vi "New Report Schema and Output Table Create.vi"() -> (0 "error out":errorcluster)   [LabVIEW 2023, in "HardwareAbstractionLayer_LVOOP.lvlib" / "Report.lvclass"]
uses:
  Report.lvclass
  Database/SQL Public VI/Control/DB Options.ctl
  <vilib>/Utility/error.llb/Trim Whitespace One-Sided.vi
  <userlib>/_OpenG.lib/array/array.llb/Filter 1D Array (String)__ogtk.vi
  Database/Database.lvclass
  Control/Action FGV.ctl
  Control/Result FGV Data.ctl
  <userlib>/_OpenG.lib/array/array.llb/openg_array.lvlib
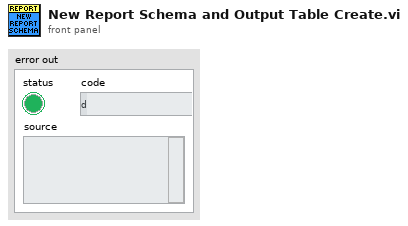
[diagram p1: front panel]
types:
  T1 = typedef "HardwareAbstractionLayer_LVOOP.lvlib/Database.lvclass/DB Options.ctl" = enum16{"Init", "Select Data", "Insert Data", "Update Data", "Delete Data", "Execute Query", "Create Schema", "Create Table", "List Tables", "List Columns", "Close"}
  T2 = typedef "HardwareAbstractionLayer_LVOOP.lvlib/Report.lvclass/Result FGV Data.ctl" = cluster{"Project Name":string, "Product Name":string, "Product Varient":string, "Test Name":string, "Test Phase":string, "Test Description":string, "Temp Chamber Name":string, "Schema":string, "Total No of Cycles":u32, "Current Cycle Number":u32, "Cycle Duration":u32, "Current Test Mode":string}
  T3 = typedef "HardwareAbstractionLayer_LVOOP.lvlib/Report.lvclass/Action FGV.ctl" = enum16{"Init", "Set Project Name", "Set Product Name", "Set Product Varient", "Set Test Name", "Set Test Phase", "Set Test Description", "Set Temp Chamber Name", "Set Cycle Duration", "Set Current Cycle Number", "Set Schema", "Set Total No Of Cycle", "Set Current Test Mode", "Set All Data", "Get All Data"}
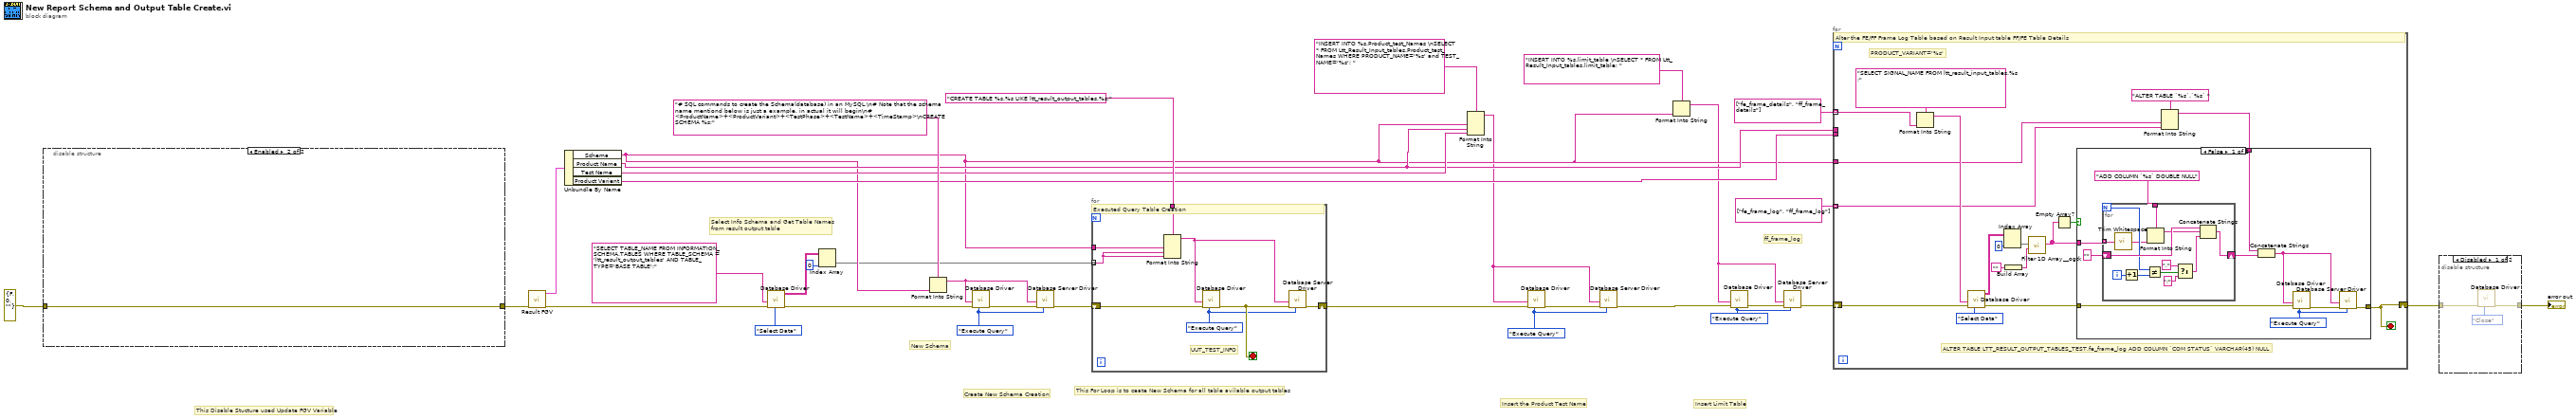
[diagram p0: block diagram]
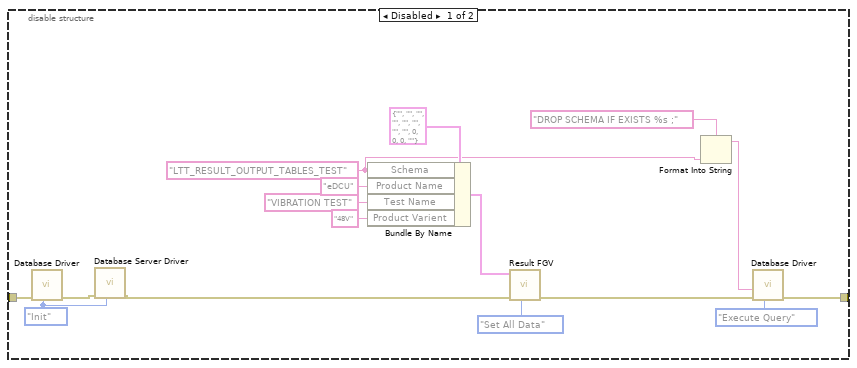
[diagram p2: hidden frame]
diagram:
  w2 = DB_Options."Execute Query" ("Options")
  w9 = DB_Options."Execute Query" ("Options")
  w5 = DB_Options."Execute Query" ("Options")
  # "This For Loop is to ceate New Schema for all table avilable output tables"
  # "ff_frame_log"
  # "Insert Limit Table"
  # "Create New Schema Creation"
  # "Select Info Schema and Get Table Names \nfrom result output table"
  # "This Disable Stucture used Update FGV Variable"
  # "Insert the Product Test Name"
  # "New Schema"
  n1 = disable-structure shown="Enabled" {
    disable-tunnel: errorcluster {"status"=FALSE, "code"=0, "source"=""} ("error in") -> [w51 w52]
    disable-tunnel: [w50 w52] -> w20
    frame Disabled {
      w37 = DB_Options."Init" ("Options")
      w39 = "LTT_RESULT_OUTPUT_TABLES_TEST" ("Schema")
      n2 = call "Database Driver.vi"("Options"=w37, "error in"=w51) -> ("error out"=w38:errorcluster)  [unwired: 6 in, 3 out]
      n3 = call "Database Server Driver.vi"("Options"=w37, "error in"=w38) -> ("error out"=w36:errorcluster)  [unwired: 6 in, 3 out]
      n4 = Bundle By Name(cluster=T2 {"Project Name"="", "Product Name"="", "Product Varient"="", "Test Name"="", "Test Phase"="", "Test Description"="", "Temp Chamber Name"="", "Schema"="", "Total No of Cycles"=0, "Current Cycle Number"=0, "Cycle Duration"=0, "Current Test Mode"=""} ("Result FGV Data In"), "Schema"=w39, "Product Name"="eDCU", "Test Name"="VIBRATION TEST", "Product Varient"="48V") -> (w47:T2)
      n5 = call "Result FGV.vi"("Action(Get All Data)"=Action_FGV."Set All Data" ("Action"), "error in"=w36, "Result FGV Data In"=w47) -> ("error out"=w43:errorcluster)  [unwired: 7 in, 1 out]
      n6 = Format Into String(format string="DROP SCHEMA IF EXISTS %s ;", w39) -> (resulting string=w40:string)  [unwired: 2 in, 1 out]
      n7 = call "Database Driver.vi"("Options"=DB_Options."Execute Query", "error in"=w43, "SQL query"=w40) -> ("error out"=w50:errorcluster)  [unwired: 5 in, 3 out]
    }
    frame Enabled {
    }
  }
  n8 = call "Result FGV.vi"("error in"=w20) -> ("error out"=w30:errorcluster, "Result FGV Data Out"=w31:T2)  [unwired: 9 in]
  n9 = Unbundle By Name(w31) -> ("Schema"=w16:string, "Product Name"=w17:string, "Test Name"=w21:string, "Product Varient"=w18:string)
  n10 = call "Database Driver.vi"("Options"=DB_Options."Select Data", "error in"=w30, "SQL query"="SELECT TABLE_NAME FROM INFORMATION_SCHEMA.TABLES WHERE TABLE_SCHEMA = 'ltt_result_output_tables' AND TABLE_TYPE='BASE TABLE';") -> ("error out"=w27:errorcluster, "data"=w25:string[][])  [unwired: 5 in, 2 out]
  n11 = Index Array(array=w25, index (col)=0 ("disabled index (col)")) -> (element=w13:string[])  [unwired: 1 in]
  n12 = Format Into String(format string="# SQL commands to create the Schema(database) in an MySQL.\n# Note that the schema name mentiond below is just a example, in actual it will begin\n# <ProductName>+<ProductVariant>+<TestPhase>+<TestName>+<TimeStamp>\nCREATE SCHEMA %s;", w16) -> (resulting string=w10:string)  [unwired: 2 in, 1 out]
  n13 = call "Database Driver.vi"("Options"=w9, "error in"=w27, "SQL query"=w10) -> ("error out"=w12:errorcluster)  [unwired: 5 in, 3 out]
  n14 = call "Database Server Driver.vi"("Options"=w9, "error in"=w12, "SQL query"=w10) -> ("error out"=w11:errorcluster)  [unwired: 5 in, 3 out]
  n15 = for {
    tunnel: w16 -> [w59]
    tunnel: "CREATE TABLE %s.%s LIKE ltt_result_output_tables.%s;" ("format string") -> [w58]
    shift-right: [w55] -> w32
    shift-left: w11 -> [w60]
    tunnel: w13 -> [w57] mode=indexing
    stop <- w56 stop-if-true
    w53 = DB_Options."Execute Query" ("Options")
    # "UUT_TEST_INFO"
    # "Executed Query Table Creation"
    n16 = Format Into String(format string=w58, w59, w57, w57) -> (resulting string=w54:string)  [unwired: 2 in, 1 out]
    n17 = call "Database Driver.vi"("Options"=w53, "error in"=w60, "SQL query"=w54) -> ("error out"=w56:errorcluster)  [unwired: 5 in, 3 out]
    n18 = call "Database Server Driver.vi"("Options"=w53, "error in"=w56, "SQL query"=w54) -> ("error out"=w55:errorcluster)  [unwired: 5 in, 3 out]
  }
  n19 = Format Into String(format string="INSERT INTO %s.Product_test_Names \nSELECT * FROM Ltt_Result_Input_tables.Product_test_Names WHERE PRODUCT_NAME='%s' and TEST_NAME='%s'; ", w16, w17, w21) -> (resulting string=w6:string)  [unwired: 2 in, 1 out]
  n20 = call "Database Driver.vi"("Options"=w5, "error in"=w32, "SQL query"=w6) -> ("error out"=w8:errorcluster)  [unwired: 5 in, 3 out]
  n21 = call "Database Server Driver.vi"("Options"=w5, "error in"=w8, "SQL query"=w6) -> ("error out"=w7:errorcluster)  [unwired: 5 in, 3 out]
  n22 = Format Into String(format string="INSERT INTO %s.limit_table \nSELECT * FROM Ltt_Result_Input_tables.limit_table; ", w16) -> (resulting string=w1:string)  [unwired: 2 in, 1 out]
  n23 = call "Database Driver.vi"("Options"=w2, "error in"=w7, "SQL query"=w1) -> ("error out"=w4:errorcluster)  [unwired: 5 in, 3 out]
  n24 = call "Database Server Driver.vi"("Options"=w2, "error in"=w4, "SQL query"=w1) -> ("error out"=w3:errorcluster)  [unwired: 5 in, 3 out]
  n25 = for {
    tunnel: w18 -> [_]
    tunnel: w17 -> [_]
    tunnel: w16 -> [w72]
    shift-right: [w66] -> w19
    shift-left: w3 -> [w77]
    tunnel: string[] ["fe_frame_details", "ff_frame_details"] -> [w71] mode=indexing
    tunnel: string[] ["fe_frame_log", "ff_frame_log"] -> [w70] mode=indexing
    stop <- w66 stop-if-true
    # "ALTER TABLE LTT_RESULT_OUTPUT_TABLES_TEST.fe_frame_log ADD COLUMN `COM STATUS` VARCHAR(45) NULL"
    # "PRODUCT_VARIANT='%s'"
    # "Alter the FE/FF Frame Log Table based on Result Input table FF/FE Table Details"
    n26 = Format Into String(format string="SELECT SIGNAL_NAME FROM ltt_result_input_tables.%s ;", w71) -> (resulting string=w76:string)  [unwired: 2 in, 1 out]
    n27 = call "Database Driver.vi"("Options"=DB_Options."Select Data", "error in"=w77, "SQL query"=w76) -> ("error out"=w68:errorcluster, "data"=w75:string[][])  [unwired: 5 in, 2 out]
    n28 = Index Array(array=w75, index (col)=0 ("disabled index (col)")) -> (element=w64:string[])  [unwired: 1 in]
    n29 = Build Array("") -> (w61:string[])
    n30 = call-poly <userlib>:"Filter 1D Array__ogtk.vi"("items to filter"=w61, "array"=w64) -> ("filtered array"=w63:string[])  [unwired: 4 in, 1 out]
    n31 = Empty Array?(array=w63) -> (empty?=w65:bool)
    n32 = Format Into String(format string="ALTER TABLE `%s`.`%s` ", w72, w70) -> (resulting string=w69:string)  [unwired: 2 in, 1 out]
    n33 = case shown="False" w65 {
      tunnel: w63 -> [w88 _]
      tunnel: w69 -> [w86 _]
      tunnel: w68 -> [w84 w102]
      tunnel: [w81 w102] -> w66
      frame False {
        w80 = DB_Options."Execute Query" ("Options")
        n34 = for {
          N -> [w92]
          tunnel: [w101] -> _ mode=indexing
          tunnel: w88 -> [w101] mode=indexing
          shift-right: [w99] -> w85
          shift-left: "" -> [w100]
          tunnel: "ADD COLUMN `%s` DOUBLE NULL" -> [w98]
          i -> [w94]
          n35 = call <vilib>:"Trim Whitespace.vi"("string"=w101) -> ("trimmed string"=w89:string)  [unwired: 1 in]
          n36 = Increment(x=w94) -> (x+1=w93:i32)
          n37 = Not Equal?(x=w92, y=w93) -> (x != y?=w91:bool)
          n38 = Format Into String(format string=w98, w89) -> (resulting string=w97:string)  [unwired: 2 in, 1 out]
          n39 = Select(t="," ("string"), s=w91, f=";") -> (s? t:f=w90:string)
          n40 = Concatenate Strings(w100, w97, w90) -> (w99:string)
        }
        n41 = Concatenate Strings(w86, w85) -> (w79:string)
        n42 = call "Database Driver.vi"("Options"=w80, "error in"=w84, "SQL query"=w79) -> ("error out"=w82:errorcluster)  [unwired: 5 in, 3 out]
        n43 = call "Database Server Driver.vi"("Options"=w80, "error in"=w82, "SQL query"=w79) -> ("error out"=w81:errorcluster)  [unwired: 5 in, 3 out]
      }
      frame True {
      }
    }
  }
  n44 = disable-structure shown="Disabled" {
    disable-tunnel: [w104 w106] -> w34
    disable-tunnel: w19 -> [w103 w106]
    frame Disabled {
      n45 = call "Database Driver.vi"("Options"=DB_Options."Close", "error in"=w103) -> ("error out"=w104:errorcluster)  [unwired: 6 in, 3 out]
    }
    frame Enabled {
    }
  }
  "error out" <- w34
